vi "Validate Routing Channel Reference.vi"(8 "error in (no error)":errorcluster, 11 "Channel Ref in":T1 format="%.0x") -> (0 "error out":errorcluster, 3 "Channel Ref out":T1 format="%.0x")   [LabVIEW 2017, in "Routing and Faulting Scripting.lvlib"]
uses:
  Routing and Faulting Scripting.lvlib
  <vilib>/NI Veristand/Custom Device API/Custom Device Item Ref.ctl
  Shared/Constants.vi
  Shared/Routing and Faulting Shared.lvlib
  <vilib>/NI Veristand/Custom Device API/Custom Device API.lvlib
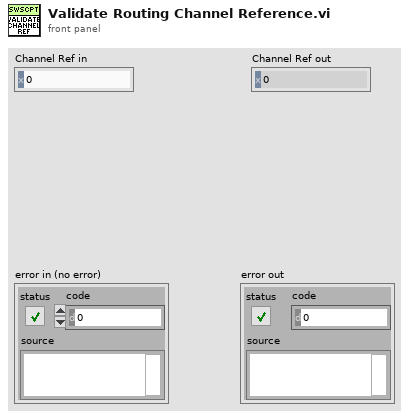
[diagram p1: front panel]
types:
  T1 = typedef "Custom Device API.lvlib/Custom Device Item Ref.ctl" = u64
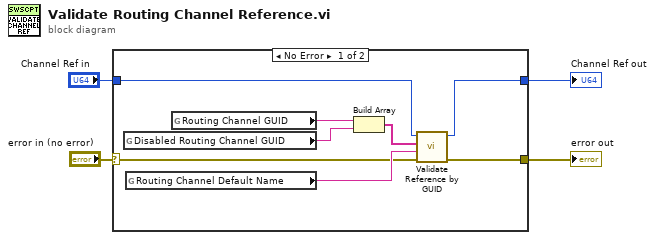
[diagram p0: block diagram]
diagram:
  n1 = case shown="No Error" "error in (no error)" {
    selector: "error in (no error)" -> [w9 w14]
    tunnel: "Channel Ref in" -> [w12 w13]
    tunnel: [w8 w14] -> w2
    tunnel: [w11 w13] -> w1
    frame No Error {
      n2 = global read "Constants.vi" "Disabled Routing Channel GUID"() -> (w6:string)
      n3 = global read "Constants.vi" "Routing Channel Default Name"() -> (w10:string)
      n4 = global read "Constants.vi" "Routing Channel GUID"() -> (w7:string)
      n5 = Build Array(w7, w6) -> (w5:string[])
      n6 = call "Validate Reference by GUID.vi"("error in (no error)"=w9, "Name"=w10, "Valid GUIDs"=w5, "Ref in"=w12) -> ("error out"=w8:errorcluster, "Ref out"=w11:T1)  [unwired: 6 in]
    }
    frame Error {
    }
  }
  "error out" <- w2
  "Channel Ref out" <- w1
